vi "READ Configurations V1.00.vi"(2 "OpenParameters(T)orDataBuffers(F)":bool, 6 "CCD Scan Parameters.INI path":path, 9 "CCD Scan Parameters.Data path":path) -> (0 "Parameters":T2={"Magnetic Field"=0.0, "Temperature"=0.0, "Exposure Time"=0.0, "Mag ID string"="Cell 12", "User Name"="Albert Einstein", "Comments"="", "SaveComments?"=1, "X-Axis Unit"=1, "Delimiter"=0, "File Format"=0, "Sample Name"="Sample1"} {"File Format" items=["Macintosh (EOL: CR)", "Unix (EOL: LF)", "DOS/Windows (EOL: CR+LF)"]; "Delimiter" items=["TAB", "COMMA", "SPACE"]; "X-Axis Unit" items=["Point #", "nm", "eV", "meV", "cm-1"]; "SaveComments?" items=["Bare data only", "Saved in the Header Area", "Saved as a Parameter File"]; "Exposure Time" format="%.2f"; "Temperature" format="%.2f"; "Magnetic Field" format="%.2f"}, 1 "Parameters#2":T3={"MaxBufferSize"=2, "Mag GPIB Address"=5, "Max Current (kA)"=36.0, "LTC-GPIB Address"="", "Temp Tolerance"=1.0} {"Temp Tolerance" format="%.2f"; "Max Current (kA)" format="%.2f"}, 3 "X-Axis Array":dbl[][](array[numeric]) format="%.2f", 4 "Data Array":dbl[][](array[numeric]) format="%.2f", 5 "Control Parameters":T1={"Grating Density"=enum."1200", "Offset"=0.0, "Save All Data in ONE file"=FALSE, "Auto Save Data"=FALSE, "Most recent saved file"=path "erererere", "Filename Prefix"="MyData", "Extension"=4, "Suffix"="", "Current Path"=path "/Volumes/DATA"} {"Extension" items=["DOS field", "\".001\",\".002\", ...", "001 (No dot)", "\".A\",\".B\", ...", "±Field", "pField nField", "Temperature", "User Defined"]; "Offset" format="%.2f"}, 7 "Background":i32[](array[numeric])=[1198, 1190, 1193, 1194, 1189, 1188, 1196, 1190, 1202, 1191, 1193, 1192, 1199, 1189, 1194, 1189, 1197, 1191, 1187, 1192, 1195, 1189, 1195, 1191, 1199, 1194, 1192, 1191, 1193, 1197, 1193, 1193, 1194, 1200, 1191, 1190, 1187, 1195, 1189, 1188, 1191, 1194, 1187, 1192, 1198, 1193, 1190, 1192, 1190, 1193, 1191, 1190, 1191, 1189, 1192, 1194, 1190, 1193, 1193, 1191, 1194, 1182, 1190, 1188, 1199, 1192, 1196, 1195, 1186, 1189, 1188, 1185, 1194, 1187, 1193, 1194, 1190, 1189, 1189, 1187, 1196, 1195, 1191, 1197, 1192, 1200, 1187, 1194, 1189, 1193, 1195, 1196, 1186, 1192, 1190, 1194, 1194, 1190, 1191, 1193, 1197, 1197, 1185, 1199, 1190, 1195, 1196, 1184, 1193, 1193, 1193, 1191, 1189, 1190, 1199, 1193, 1191, 1194, 1191, 1192, 1186, 1190, 1194, 1189, 1194, 1190, 1191, 1192, 1192, 1196, 1192, 1192, 1189, 1193, 1198, 1186, 1191, 1193, 1187, 1194, 1190, 1190, 1191, 1189, 1194, 1195, 1189, 1192, 1185, 1193, 1192, 1192, 1189, 1191, 1191, 1190, 1196, 1194, 1193, 1191, 1189, 1191, 1196, 1192, 1192, 1189, 1196, 1191, 1193, 1192, 1188, 1190, 1194, 1192, 1185, 1191, 1194, 1191, 1189, 1195, 1192, 1196, 1190, 1193, 1191, 1189, 1194, 1195, 1191, 1187, 1190, 1196, 1196, 1192, 1197, 1191, 1189, 1192, 1192, 1200, 1192, 1193, 1190, 1192, 1187, 1198, 1186, 1196, 1201, 1199, 1200, 1191, 1196, 1200, 1192, 1191, 1193, 1185, 1192, 1194, 1186, 1190, 1188, 1189, 1201, 1197, 1191, 1194, 1193, 1194, 1195, 1198, 1200, 1192, 1192, 1193, 1193, 1195, 1187, 1193, 1192, 1187, 1189, 1186, 1191, 1197, 1191, 1200, 1194, 1192, 1187, 1196, 1191, 1191, 1196, 1187, 1190, 1193, 1189, 1193, 1190, 1188, 1188, 1190, 1197, 1188, 1191, 1195, 1188, 1191, 1188, 1194, 1193, 1187, 1200, 1192, 1197, 1190, 1196, 1200, 1191, 1189, 1193, 1189, 1186, 1196, 1185, 1198, 1195, 1186, 1191, 1197, 1191, 1193, 1195, 1193, 1191, 1198, 1189, 1183, 1200, 1197, 1192, 1192, 1192, 1196, 1191, 1190, 1194, 1188, 1198, 1193, 1195, 1190, 1187, 1192, 1191, 1195, 1188, 1190, 1191, 1187, 1189, 1185, 1189, 1196, 1198, 1191, 1190, 1196, 1197, 1193, 1187, 1186, 1195, 1191, 1193, 1192, 1196, 1190, 1192, 1192, 1192, 1190, 1195, 1192, 1191, 1193, 1197, 1184, 1190, 1188, 1192, 1194, 1190, 1193, 1195, 1195, 1194, 1189, 1193, 1191, 1194, 1186, 1189, 1192, 1191, 1182, 1190, 1197, 1194, 1188, 1193, 1191, 1186, 1194, 1197, 1193, 1191, 1187, 1194, 1194, 1191, 1189, 1195, 1194, 1189, 1196, 1187, 1186, 1192, 1194, 1196, 1191, 1193, 1191, 1188, 1190, 1199, 1198, 1196, 1196, 1190, 1194, 1191, 1194, 1187, 1195, 1190, 1194, 1196, 1194, 1189, 1193, 1189, 1194, 1189, 1195, 1192, 1194, 1193, 1191, 1197, 1187, 1189, 1189, 1188, 1197, 1192, 1189, 1193, 1194, 1183, 1202, 1187, 1192, 1184, 1188, 1186, 1193, 1189, 1195, 1189, 1193, 1197, 1189, 1194, 1191, 1194, 1192, 1191, 1191, 1196, 1194, 1190, 1193, 1192, 1195, 1197, 1198, 1193, 1202, 1196, 1194, 1194, 1190, 1193, 1190, 1195, 1192, 1187, 1194, 1197, 1190, 1194, 1189, 1198, 1192, 1191, 1192, 1192, 1191, 1191, 1193, 1191, 1191, 1198, 1186, 1192, 1185, 1185, 1188, 1194, 1196, 1194, 1195, 1190, 1194, 1191, 1190, 1195, 1191, 1191, 1195, 1192, 1194, 1201, 1187, 1191, 1195, 1187, 1192, 1192, 1193, 1200, 1188, 1189, 1189, 1197, 1189, 1188, 1197, 1195, 1191, 1189, 1190, 1195, 1189, 1191, 1194, 1186, 1192, 1190, 1191, 1188, 1195, 1192, 1191, 1191, 1199, 1190, 1190, 1190, 1192, 1187, 1193, 1197, 1197, 1186, 1193, 1189, 1192, 1197, 1184, 1187, 1188, 1192, 1192, 1192, 1189, 1192, 1190, 1194, 1191, 1186, 1196, 1194, 1189, 1193, 1191, 1186, 1189, 1193, 1195, 1196, 1197, 1199, 1194, 1190, 1193, 1194, 1190, 1198, 1196, 1194, 1195, 1194, 1184, 1188, 1195, 1197, 1190, 1194, 1190, 1191, 1195, 1198, 1188, 1193, 1194, 1195, 1198, 1195, 1191, 1197, 1192, 1198, 1190, 1196, 1191, 1194, 1188, 1189, 1198, 1192, 1198, 1195, 1185, 1191, 1193, 1192, 1197, 1195, 1195, 1195, 1193, 1190, 1190, 1190, 1198, 1195, 1191, 1194, 1190, 1190, 1194, 1194, 1195, 1192, 1190, 1194, 1195, 1192, 1192, 1194, 1189, 1192, 1193, 1188, 1194, 1195, 1196, 1193, 1192, 1201, 1191, 1198, 1197, 1191, 1192, 1191, 1194, 1193, 1188, 1192, 1189, 1183, 1189, 1190, 1192, 1189, 1196, 1193, 1197, 1185, 1193, 1189, 1191, 1196, 1195, 1193, 1193, 1191, 1189, 1193, 1192, 1192, 1192, 1190, 1191, 1193, 1193, 1197, 1195, 1189, 1193, 1188, 1194, 1197, 1194, 1195, 1196, 1190, 1194, 1188, 1197, 1195, 1191, 1195, 1192, 1194, 1188, 1190, 1197, 1197, 1191, 1187, 1197, 1191, 1193, 1188, 1191, 1194, 1193, 1195, 1192, 1195, 1189, 1193, 1193, 1195, 1190, 1192, 1196, 1188, 1187, 1193, 1192, 1192, 1194, 1185, 1199, 1190, 1193, 1191, 1198, 1189, 1190, 1191, 1190, 1193, 1195, 1186, 1190, 1193, 1191, 1189, 1197, 1193, 1198, 1190, 1192, 1193, 1191, 1196, 1193, 1196, 1190, 1190, 1198, 1192, 1199, 1198, 1190, 1191, 1191, 1196, 1190, 1196, 1195, 1191, 1196, 1195, 1193, 1190, 1190, 1195, 1193, 1187, 1197, 1185, 1191, 1189, 1191, 1193, 1192, 1188, 1196, 1193, 1191, 1193, 1193, 1190, 1192, 1192, 1192, 1195, 1191, 1195, 1189, 1189, 1191, 1191, 1185, 1192, 1191, 1193, 1201, 1199, 1197, 1206, 1201, 1207, 1200, 1198, 1195, 1188, 1194, 1186, 1190, 1197, 1188, 1193, 1196, 1193, 1192, 1192, 1188, 1196, 1186, 1193, 1194, 1188, 1190, 1190, 1192, 1190, 1191, 1191, 1200, 1192, 1199, 1193, 1190, 1190, 1199, 1187, 1193, 1190, 1188, 1194, 1194, 1196, 1194, 1195, 1190, 1187, 1187, 1196, 1193, 1199, 1190, 1193, 1193, 1191, 1198, 1192, 1193, 1192, 1193, 1189, 1189, 1197, 1189, 1194, 1193, 1192, 1185, 1198, 1193, 1189, 1192, 1193, 1196, 1190, 1195, 1189, 1196, 1198, 1190, 1191, 1193, 1186, 1189, 1195, 1188, 1197, 1188, 1191, 1185, 1190, 1193, 1188, 1198, 1192, 1193, 1194, 1194, 1189, 1184, 1193, 1199, 1193, 1192, 1193, 1190, 1196, 1191, 1192, 1189, 1194, 1188, 1189, 1190, 1190, 1192, 1195, 1188, 1190, 1192, 1189, 1197, 1192, 1194, 1187, 1196, 1192, 1194, 1185, 1187, 1187, 1191, 1195, 1190, 1186, 1183, 1194, 1194, 1192, 1192, 1188, 1193, 1195, 1189, 1190, 1191, 1192, 1196, 1186, 1195, 1191, 1185, 1191, 1187, 1190, 1188, 1189, 1187, 1196, 1191, 1190, 1191, 1190, 1196, 1195, 1186, 1187, 1187, 1188, 1194, 1192, 1192, 1192, 1189, 1192, 1191, 1188, 1188, 1187, 1187, 1190, 1186, 1191, 1195, 1192, 1196, 1193, 1192, 1191, 1189, 1187, 1193, 1188, 1189, 1194, 1191, 1185, 1193, 1191, 1196, 1196, 1199, 1195, 1211], 8 "FieldRamp Parameters":dbl[][](array[numeric])=[[0.0, 30.0, 1.0, 400.0], [30.0, 0.0, -1.0, 400.0], [0.0, -30.0, -1.0, 400.0], [-30.0, 0.0, 1.0, 400.0], [0.0, 30.0, 0.5, 200.0], [30.0, 0.0, -0.5, 200.0]] step=1.0 format="%.2f")   [LabVIEW 2025]
doc: "Author: Scott Hannahs <sth@magnet.fsu.edu>\n\nThis software is licensed for use under the “MIT License\"\nCopyright (c) 2025 Scott Hannahs, sth@sth@magnet.sthnet.net\n\nPermission is hereby granted, free of charge, to any person obtaining a copy of this software and associated documentation files (the \"Software\"), to deal in the Software without restriction, including without limitation the rights to use, copy, modify, merge, publish, distribute, sublicense, and/or sell copies of the Software, and to permit persons to whom the Software is furnished to do so, subject to the following conditions: The above copyright notice and this permission notice shall be included in all copies or substantial portions of the Software.\n\nTHE SOFTWARE IS PROVIDED \"AS IS\", WITHOUT WARRANTY OF ANY KIND, EXPRESS OR IMPLIED, INCLUDING BUT NOT LIMITED TO THE WARRANTIES OF MERCHANTABILITY, FITNESS FOR A PARTICULAR PURPOSE AND NONINFRINGEMENT. IN NO EVENT SHALL THE AUTHORS OR COPYRIGHT HOLDERS BE LIABLE FOR ANY CLAIM, DAMAGES OR OTHER LIABILITY, WHETHER IN AN ACTION OF CONTRACT, TORT OR OTHERWISE, ARISING FROM, OUT OF OR IN CONNECTION WITH THE SOFTWARE OR THE USE OR OTHER DEALINGS IN THE SOFTWARE."
uses:
  Parameters#2.ctl
  Parameters#1.ctl
  Parameters_Control.ctl
  <vilib>/Utility/config.llb/Read Key (String).vi
  <vilib>/Utility/config.llb/Read Key (U32).vi
  <vilib>/Utility/config.llb/Read Key (Double).vi
  <vilib>/Utility/config.llb/Read Key (Boolean).vi
  <vilib>/Utility/config.llb/Read Key (Path).vi
  <vilib>/Utility/config.llb/NI_LVConfig.lvlib
panel:
  out "Temperature array":sgl[](array[numeric]) format="%.3f"
  out "Field array":sgl[](array[numeric]) format="%.3f"
  out "2D Y-array":sgl[][](array[numeric]) format="%.3f"
  out "2D X-array":sgl[][](array[numeric]) format="%.3f"
  out "error out":errorcluster
  out "found?":bool
  out "Buffer Size":i32[](array[numeric])
  out "FieldRampSize":i32[](array[numeric])
  out "X-size":i32[](array[numeric])
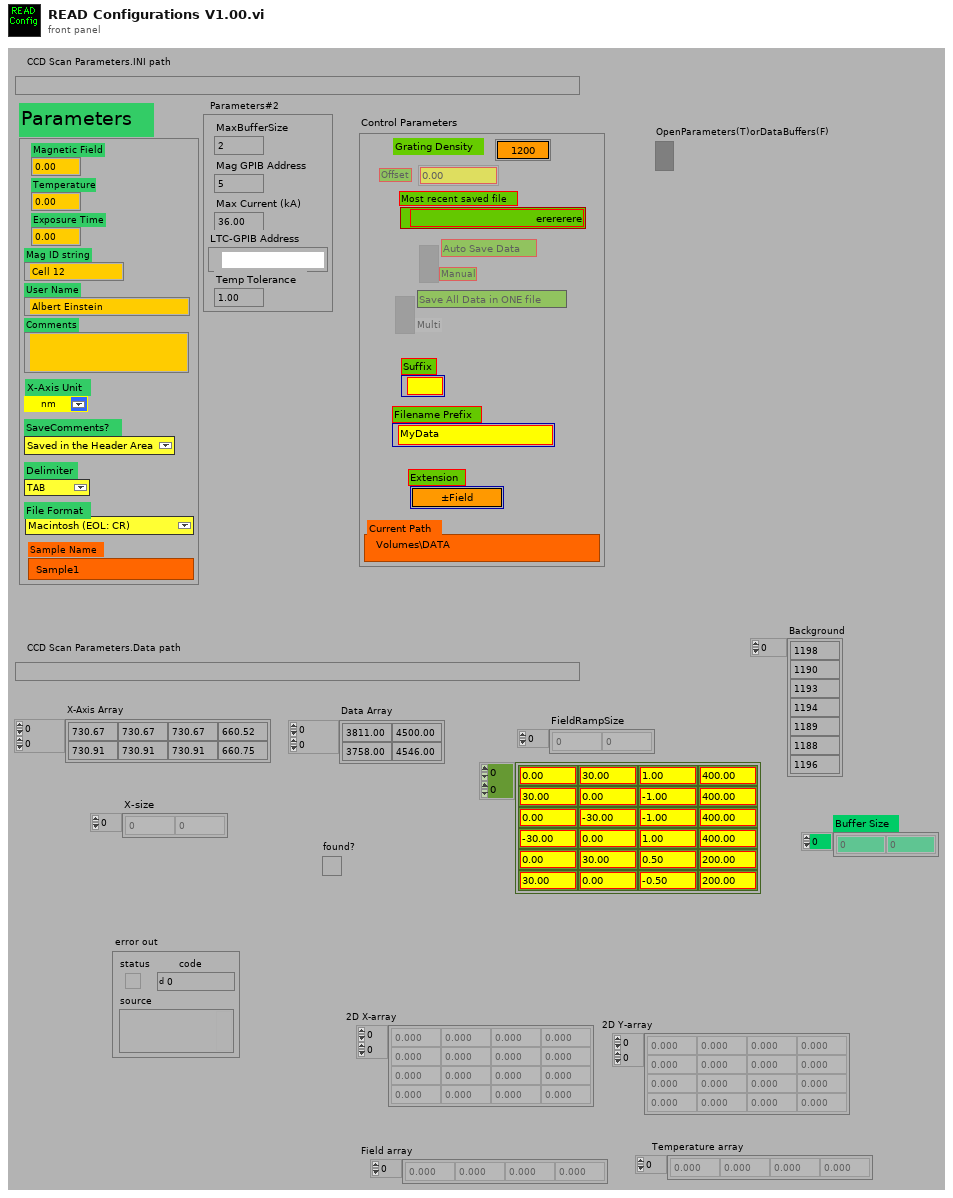
[diagram p1: front panel]
types:
  T1 = typedef "Parameters_Control.ctl" = cluster{"Grating Density":enum16{"150", "300", "600", "1200", "1800"}, "Offset":dbl, "Save All Data in ONE file":bool, "Auto Save Data":bool, "Most recent saved file":path, "Filename Prefix":string, "Extension":u16, "Suffix":string, "Current Path":path}
  T2 = typedef "Parameters#1.ctl" = cluster{"Magnetic Field":dbl, "Temperature":dbl, "Exposure Time":dbl, "Mag ID string":string, "User Name":string, "Comments":string, "SaveComments?":u16, "X-Axis Unit":u16, "Delimiter":u16, "File Format":u16, "Sample Name":string}
  T3 = typedef "Parameters#2.ctl" = cluster{"MaxBufferSize":i32, "Mag GPIB Address":i32, "Max Current (kA)":dbl, "LTC-GPIB Address":refnum<visa-resource-name>, "Temp Tolerance":dbl}
  T4 = typedef "NI_LVConfig.lvlib/Config Data RefNum.ctl" = refnum<k1>
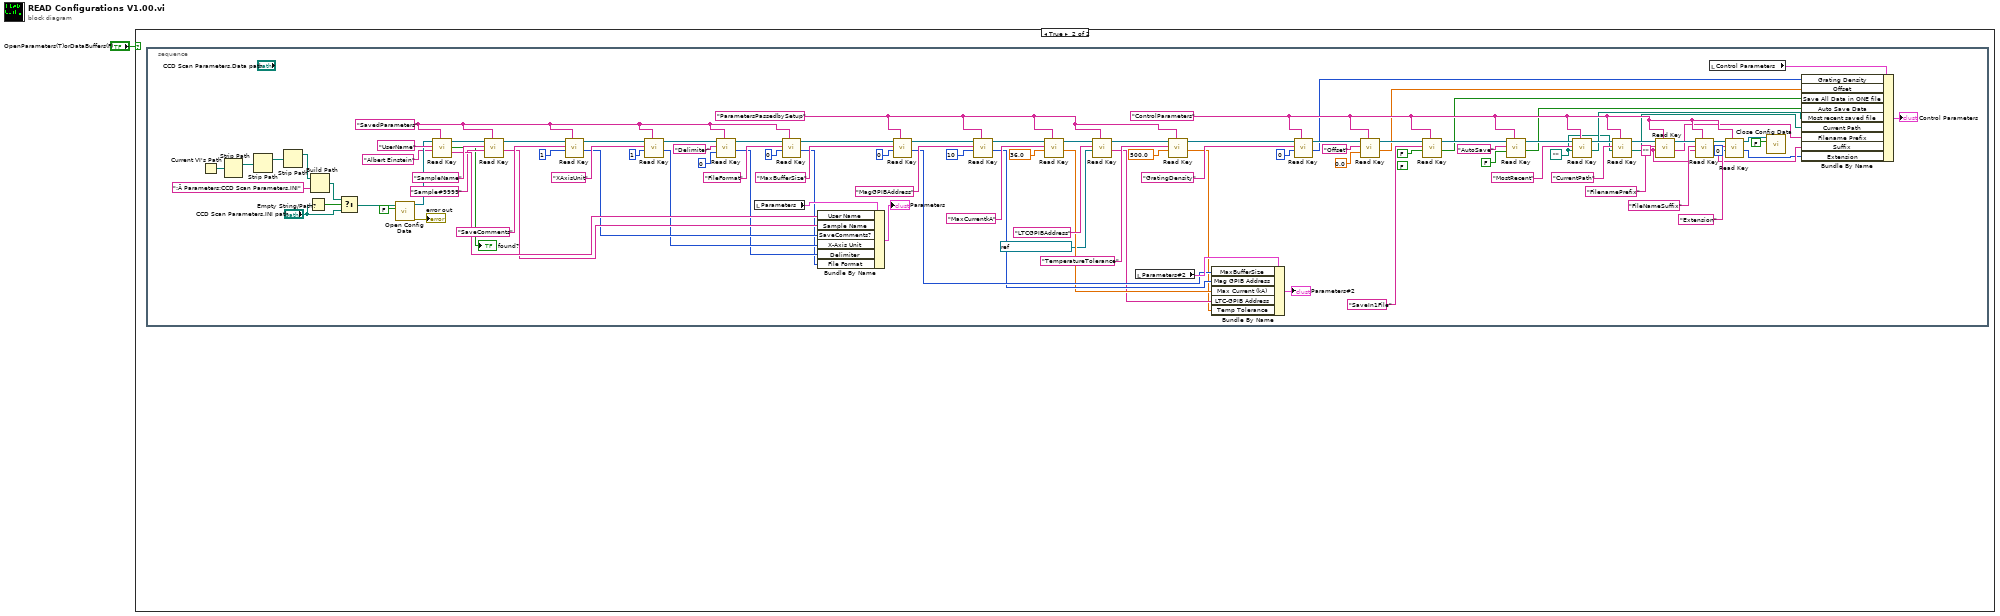
[diagram p0: block diagram]
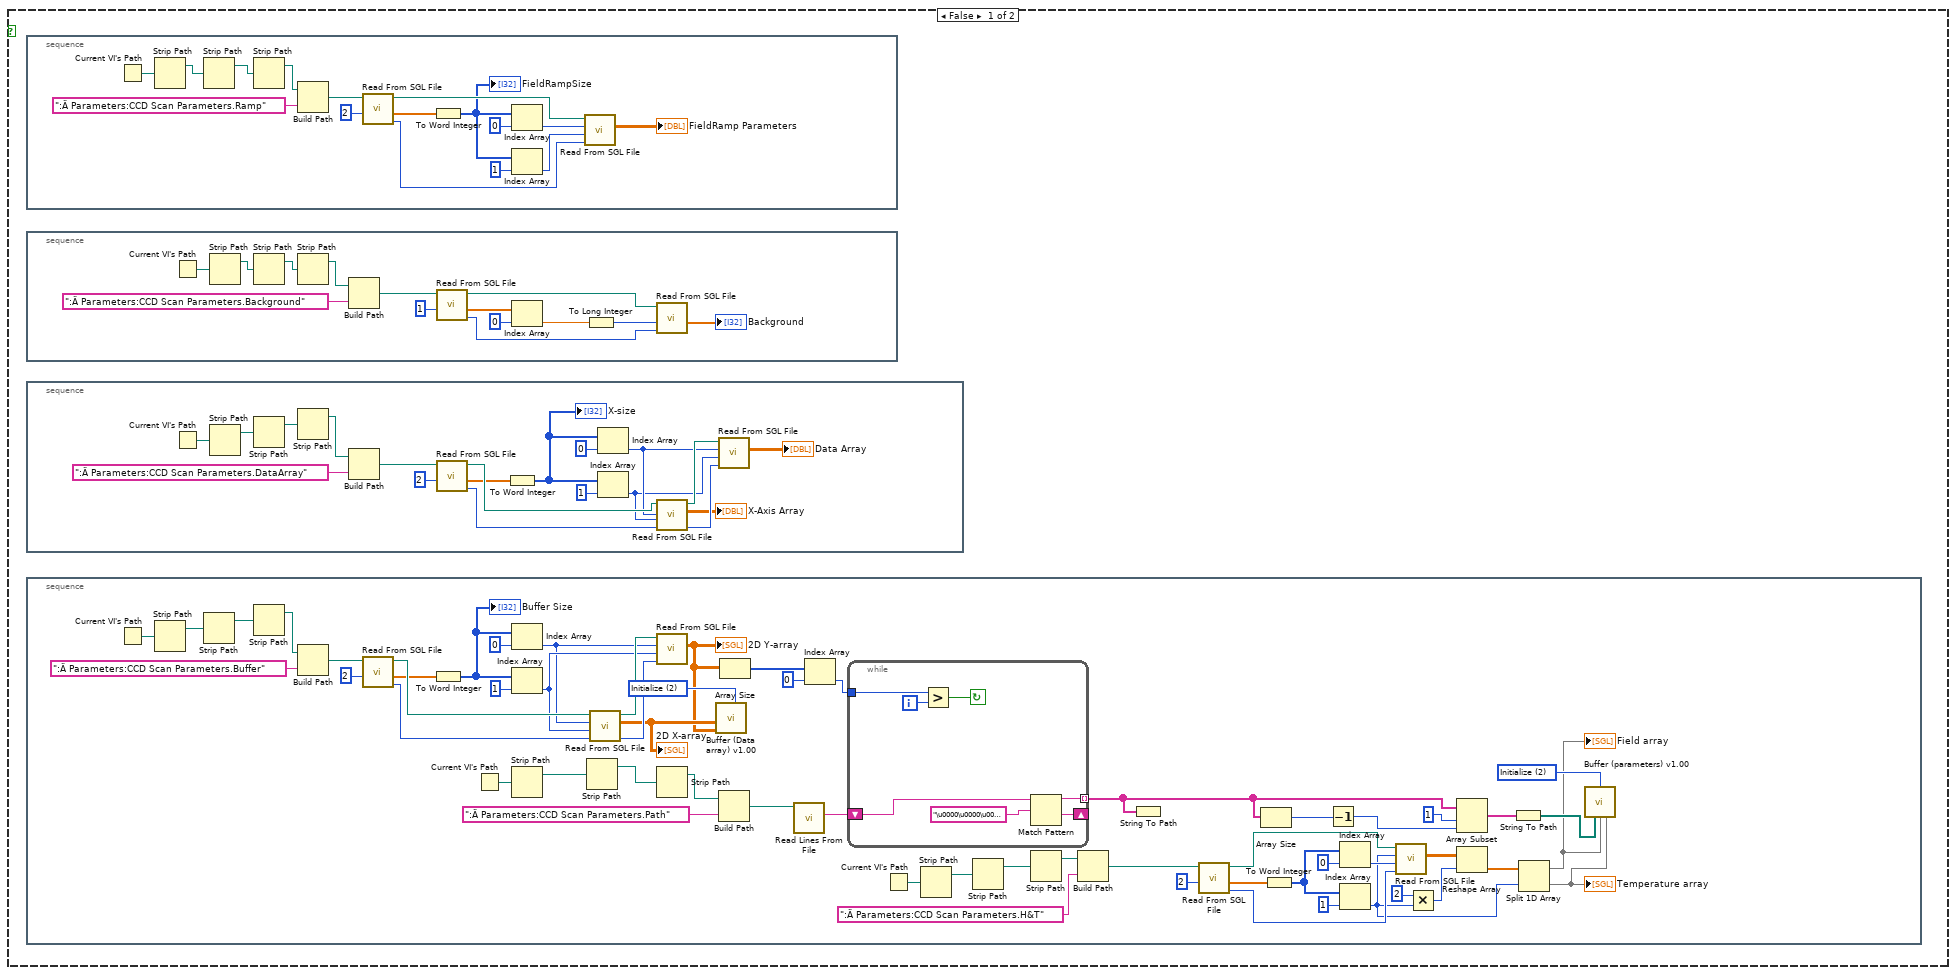
[diagram p2: hidden frame]
diagram:
  n1 = case shown="True" "OpenParameters(T)orDataBuffers(F)" {
    frame False {
      n2 = stacked-sequence {
        frame #0 {
          n3 = Current VI's Path() -> (path=w18:path)
          n4 = Strip Path(path=w18) -> (stripped path=w22:path)  [unwired: 1 out]
          n5 = Strip Path(path=w22) -> (stripped path=w21:path)  [unwired: 1 out]
          n6 = Strip Path(path=w21) -> (stripped path=w19:path)  [unwired: 1 out]
          n7 = Build Path(base path=w19, name or relative path=":Ä Parameters:CCD Scan Parameters.Ramp") -> (appended path=w17:path)
          n8 = call <vilib>:"Read From SGL File.vi"("2D number of columns/1D count (all as 1D: -1)"=2, "file path (dialog if empty)"=w17) -> ("mark after read (bytes)"=w30:i32, "1D array"=w26:sgl[], "new file path (Not A Path if cancelled)"=w31:path)  [unwired: 5 in, 2 out]
          n9 = To Word Integer(number=w26) -> (16bit integer=w23:i16[])
          "FieldRampSize" <- w23
          n10 = Index Array(array=w23, index=0) -> (element=w25:i16)
          n11 = Index Array(array=w23, index=1) -> (element=w24:i16)
          n12 = call <vilib>:"Read From SGL File.vi"("start of read offset (bytes:0)"=w30, "2D number of columns/1D count (all as 1D: -1)"=w24, "2D number of rows"=w25, "file path (dialog if empty)"=w31) -> ("2D array"=→"FieldRamp Parameters":sgl[][])  [unwired: 3 in, 4 out]
        }
      }
      n13 = stacked-sequence {
        frame #0 {
          n14 = Current VI's Path() -> (path=w3:path)
          n15 = Strip Path(path=w3) -> (stripped path=w7:path)  [unwired: 1 out]
          n16 = Strip Path(path=w7) -> (stripped path=w6:path)  [unwired: 1 out]
          n17 = Strip Path(path=w6) -> (stripped path=w4:path)  [unwired: 1 out]
          n18 = Build Path(base path=w4, name or relative path=":Ä Parameters:CCD Scan Parameters.Background") -> (appended path=w2:path)
          n19 = call <vilib>:"Read From SGL File.vi"("2D number of columns/1D count (all as 1D: -1)"=1, "file path (dialog if empty)"=w2) -> ("mark after read (bytes)"=w12:i32, "1D array"=w14:sgl[], "new file path (Not A Path if cancelled)"=w11:path)  [unwired: 5 in, 2 out]
          n20 = Index Array(array=w14, index=0) -> (element=w10:sgl)
          n21 = To Long Integer(number=w10) -> (32bit integer=w9:i32)
          n22 = call <vilib>:"Read From SGL File.vi"("start of read offset (bytes:0)"=w12, "2D number of columns/1D count (all as 1D: -1)"=w9, "file path (dialog if empty)"=w11) -> ("1D array"=→"Background":sgl[])  [unwired: 4 in, 4 out]
        }
      }
      n23 = stacked-sequence {
        frame #0 {
          n24 = Current VI's Path() -> (path=w46:path)
          n25 = Strip Path(path=w46) -> (stripped path=w50:path)  [unwired: 1 out]
          n26 = Strip Path(path=w50) -> (stripped path=w49:path)  [unwired: 1 out]
          n27 = Strip Path(path=w49) -> (stripped path=w47:path)  [unwired: 1 out]
          n28 = Build Path(base path=w47, name or relative path=":Ä Parameters:CCD Scan Parameters.DataArray") -> (appended path=w32:path)
          n29 = call <vilib>:"Read From SGL File.vi"("2D number of columns/1D count (all as 1D: -1)"=2, "file path (dialog if empty)"=w32) -> ("mark after read (bytes)"=w43:i32, "1D array"=w40:sgl[], "new file path (Not A Path if cancelled)"=w44:path)  [unwired: 5 in, 2 out]
          n30 = To Word Integer(number=w40) -> (16bit integer=w33:i16[])
          "X-size" <- w33
          n31 = Index Array(array=w33, index=0) -> (element=w36:i16)
          n32 = Index Array(array=w33, index=1) -> (element=w35:i16)
          n33 = call <vilib>:"Read From SGL File.vi"("start of read offset (bytes:0)"=w43, "2D number of columns/1D count (all as 1D: -1)"=w35, "2D number of rows"=w36, "file path (dialog if empty)"=w44) -> ("mark after read (bytes)"=w42:i32, "2D array"=→"X-Axis Array":sgl[][], "new file path (Not A Path if cancelled)"=w45:path)  [unwired: 3 in, 2 out]
          n34 = call <vilib>:"Read From SGL File.vi"("start of read offset (bytes:0)"=w42, "2D number of columns/1D count (all as 1D: -1)"=w35, "2D number of rows"=w36, "file path (dialog if empty)"=w45) -> ("2D array"=→"Data Array":sgl[][])  [unwired: 3 in, 4 out]
        }
      }
      n35 = stacked-sequence {
        frame #0 {
          w96 = u16 2 items=["Read", "Write", "Initialize"] ("Read(0) or Write(1)")
          w99 = u16 2 items=["Read", "Write", "Initialize"] ("Read(0) or Write(1)")
          n36 = Current VI's Path() -> (path=w80:path)
          n37 = Strip Path(path=w80) -> (stripped path=w84:path)  [unwired: 1 out]
          n38 = Strip Path(path=w84) -> (stripped path=w83:path)  [unwired: 1 out]
          n39 = Strip Path(path=w83) -> (stripped path=w81:path)  [unwired: 1 out]
          n40 = Build Path(base path=w81, name or relative path=":Ä Parameters:CCD Scan Parameters.Buffer") -> (appended path=w79:path)
          n41 = call <vilib>:"Read From SGL File.vi"("2D number of columns/1D count (all as 1D: -1)"=2, "file path (dialog if empty)"=w79) -> ("mark after read (bytes)"=w106:i32, "1D array"=w101:sgl[], "new file path (Not A Path if cancelled)"=w108:path)  [unwired: 5 in, 2 out]
          n42 = To Word Integer(number=w101) -> (16bit integer=w97:i16[])
          "Buffer Size" <- w97
          n43 = Current VI's Path() -> (path=w91:path)
          n44 = Index Array(array=w97, index=0) -> (element=w73:i16)
          n45 = Index Array(array=w97, index=1) -> (element=w100:i16)
          n46 = Strip Path(path=w91) -> (stripped path=w95:path)  [unwired: 1 out]
          n47 = Strip Path(path=w95) -> (stripped path=w94:path)  [unwired: 1 out]
          n48 = call <vilib>:"Read From SGL File.vi"("start of read offset (bytes:0)"=w106, "2D number of columns/1D count (all as 1D: -1)"=w100, "2D number of rows"=w73, "file path (dialog if empty)"=w108) -> ("mark after read (bytes)"=w105:i32, "2D array"=w98:sgl[][], "new file path (Not A Path if cancelled)"=w107:path)  [unwired: 3 in, 2 out]
          "2D X-array" <- w98
          n49 = call <vilib>:"Read From SGL File.vi"("start of read offset (bytes:0)"=w105, "2D number of columns/1D count (all as 1D: -1)"=w100, "2D number of rows"=w73, "file path (dialog if empty)"=w107) -> ("2D array"=w63:sgl[][])  [unwired: 3 in, 4 out]
          "2D Y-array" <- w63
          n50 = Strip Path(path=w94) -> (stripped path=w92:path)  [unwired: 1 out]
          n51 = call "Buffer (Data array) v1.00.vi"("Action"=w99, "Y-Buffer input"=w63, "X-Buffer input"=w98) -> ()  [unwired: 5 in, 4 out]
          n52 = Build Path(base path=w92, name or relative path=":Ä Parameters:CCD Scan Parameters.Path") -> (appended path=w90:path)
          n53 = Array Size(array=w63) -> (size(s)=w62:i32[])
          n54 = call <vilib>:"Read Lines From File.vi"("file path (dialog if empty)"=w90) -> ("line string"=w89:string)  [unwired: 5 in, 3 out]
          n55 = Index Array(array=w62, index=0 ("Index")) -> (element=w58:i32)
          n56 = while {
            tunnel: w58 -> [w109]
            tunnel: [w112] -> w60 mode=indexing
            shift-left: w89 -> [w114]
            shift-right: [w113] -> _
            i -> [w110]
            stop <- w111 continue-if-true
            n57 = Greater?(x=w109, y=w110) -> (0:w111:bool)
            n58 = Match Pattern(string=w114, regular expression="\u0000\u0000\u0000\u001d") -> (before substring=w112:string, after substring=w113:string)  [unwired: 1 in, 2 out]
          }
          n59 = Current VI's Path() -> (path=w75:path)
          n60 = Strip Path(path=w75) -> (stripped path=w78:path)  [unwired: 1 out]
          n61 = Strip Path(path=w78) -> (stripped path=w77:path)  [unwired: 1 out]
          n62 = Strip Path(path=w77) -> (stripped path=w76:path)  [unwired: 1 out]
          n63 = Build Path(base path=w76, name or relative path=":Ä Parameters:CCD Scan Parameters.H&T") -> (appended path=w67:path)
          n64 = String To Path(string=w60) -> ()  [unwired: 1 out]
          n65 = call <vilib>:"Read From SGL File.vi"("2D number of columns/1D count (all as 1D: -1)"=2, "file path (dialog if empty)"=w67) -> ("mark after read (bytes)"=w65:i32, "1D array"=w69:sgl[], "new file path (Not A Path if cancelled)"=w66:path)  [unwired: 5 in, 2 out]
          n66 = Array Size(array=w60) -> (size(s)=w86:i32)
          n67 = To Word Integer(number=w69) -> (16bit integer=w68:i16[])
          n68 = Decrement(x=w86) -> (x-1=w88:i32)
          n69 = Index Array(array=w68, index=0) -> (element=w64:i16)
          n70 = Index Array(array=w68, index=1) -> (element=w51:i16)
          n71 = call <vilib>:"Read From SGL File.vi"("start of read offset (bytes:0)"=w65, "2D number of columns/1D count (all as 1D: -1)"=w64, "2D number of rows"=w51, "file path (dialog if empty)"=w66) -> ("2D array"=w57:sgl[][])  [unwired: 3 in, 4 out]
          n72 = Multiply(x=i16 2, y=w51) -> (x*y=w55:i16)
          n73 = Array Subset(array=w60, index=1, length=w88) -> (w85:string[])
          n74 = Reshape Array(w57, w55) -> (w54:sgl[])
          n75 = String To Path(string=w85) -> (path=w59:path[])
          n76 = Split 1D Array(array=w54, index=w51) -> (first subarray=w53:sgl[], second subarray=w52:sgl[])
          "Field array" <- w53
          "Temperature array" <- w52
          n77 = call "Buffer (parameters) v1.00.vi"("Action"=w96, "FilePath Buffer in"=w59, "Field Buffer in"=w53, "Temperature Buffer in"=w52) -> ()  [unwired: 7 in, 5 out]
        }
      }
    }
    frame True {
      n78 = stacked-sequence {
        frame #0 {
          w117 = "" ("default value")
          w118 = path "" ("default value")
          (unwired) FALSE ("write configuration file? (T)")
          w163 = "ControlParameters" ("section")
          w185 = "ParametersPassedbySetup" ("section")
          w196 = "SavedParameters" ("section")
          n79 = Current VI's Path() -> (path=w210:path)
          n80 = Strip Path(path=w210) -> (stripped path=w215:path)  [unwired: 1 out]
          n81 = Strip Path(path=w215) -> (stripped path=w214:path)  [unwired: 1 out]
          n82 = Strip Path(path=w214) -> (stripped path=w211:path)  [unwired: 1 out]
          n83 = Empty String/Path?(string/path="CCD Scan Parameters.INI path") -> (empty?=w216:bool)
          n84 = Build Path(base path=w211, name or relative path=":Ä Parameters:CCD Scan Parameters.INI") -> (appended path=w209:path)
          n85 = Select(t=w209, s=w216, f="CCD Scan Parameters.INI path") -> (s? t:f=w208:path)
          n86 = call <vilib>:"Open Config Data.vi"("create file if necessary (T)"=FALSE ("create file if necessary? (T)"), "configuration file path"=w208) -> ("error out"=→"error out":errorcluster, "refnum"=w184:T4)  [unwired: 7 in, 1 out]
          n87 = call-poly <vilib>:"Read Key.vi"("section"=w196, "default value"="Albert Einstein", "key"="UserName", "refnum"=w184) -> ("value"=w160:string, "found?"=→"found?":bool, "refnum out"=w199:T4)  [unwired: 4 in, 1 out]
          n88 = call-poly <vilib>:"Read Key.vi"("section"=w196, "default value"="Sample#9999", "key"="SampleName", "refnum"=w199) -> ("value"=w159:string, "refnum out"=w198:T4)  [unwired: 4 in, 2 out]
          n89 = call-poly <vilib>:"Read Key.vi"("section"=w196, "default value"=u32 1, "key"="SaveComments", "refnum"=w198) -> ("value"=w158:u32, "refnum out"=w205:T4)  [unwired: 4 in, 2 out]
          n90 = call-poly <vilib>:"Read Key.vi"("section"=w196, "default value"=u32 1, "key"="XAxisUnit", "refnum"=w205) -> ("value"=w157:u32, "refnum out"=w203:T4)  [unwired: 4 in, 2 out]
          n91 = call-poly <vilib>:"Read Key.vi"("section"=w196, "default value"=u32 0, "key"="Delimiter", "refnum"=w203) -> ("value"=w156:u32, "refnum out"=w202:T4)  [unwired: 4 in, 2 out]
          n92 = local read "Parameters"() -> (w161:T2)
          n93 = call-poly <vilib>:"Read Key.vi"("section"=w196, "default value"=u32 0, "key"="FileFormat", "refnum"=w202) -> ("value"=w155:u32, "refnum out"=w195:T4)  [unwired: 4 in, 2 out]
          n94 = Bundle By Name(cluster=w161, "User Name"=w160, "Sample Name"=w159, "SaveComments?"=w158, "X-Axis Unit"=w157, "Delimiter"=w156, "File Format"=w155) -> (→"Parameters":T2)
          n95 = call-poly <vilib>:"Read Key.vi"("section"=w185, "default value"=u32 0, "key"="MaxBufferSize", "refnum"=w195) -> ("value"=w146:u32, "refnum out"=w194:T4)  [unwired: 4 in, 2 out]
          n96 = call-poly <vilib>:"Read Key.vi"("section"=w185, "default value"=u32 10, "key"="MagGPIBAddress", "refnum"=w194) -> ("value"=w145:u32, "refnum out"=w193:T4)  [unwired: 4 in, 2 out]
          n97 = call-poly <vilib>:"Read Key.vi"("section"=w185, "default value"=36.0, "key"="MaxCurrentkA", "refnum"=w193) -> ("value"=w144:dbl, "refnum out"=w192:T4)  [unwired: 4 in, 2 out]
          n98 = call-poly <vilib>:"Read Key.vi"("section"=w185, "default value"=refnum<visa-resource-name> "GPIB0::15::INSTR" ("VISA resource name"), "key"="LTCGPIBAddress", "refnum"=w192) -> ("value"=w143:string, "refnum out"=w191:T4)  [unwired: 4 in, 2 out]
          n99 = local read "Parameters#2"() -> (w148:T3)
          n100 = call-poly <vilib>:"Read Key.vi"("section"=w185, "default value"=500.0, "key"="TemperatureTolerance", "refnum"=w191) -> ("value"=w142:dbl, "refnum out"=w183:T4)  [unwired: 4 in, 2 out]
          n101 = Bundle By Name(cluster=w148, "MaxBufferSize"=w146, "Mag GPIB Address"=w145, "Max Current (kA)"=w144, "LTC-GPIB Address"=w143, "Temp Tolerance"=w142) -> (→"Parameters#2":T3)
          n102 = call-poly <vilib>:"Read Key.vi"("section"=w163, "default value"=u32 0, "key"="GratingDensity", "refnum"=w183) -> ("value"=w136:u32, "refnum out"=w182:T4)  [unwired: 4 in, 2 out]
          n103 = call-poly <vilib>:"Read Key.vi"("section"=w163, "default value"=0.0, "key"="Offset", "refnum"=w182) -> ("value"=w135:dbl, "refnum out"=w181:T4)  [unwired: 4 in, 2 out]
          n104 = call-poly <vilib>:"Read Key.vi"("section"=w163, "default value"=FALSE, "key"="SaveIn1File", "refnum"=w181) -> ("value"=w134:bool, "refnum out"=w180:T4)  [unwired: 4 in, 2 out]
          n105 = call-poly <vilib>:"Read Key.vi"("section"=w163, "default value"=FALSE, "key"="AutoSave", "refnum"=w180) -> ("value"=w133:bool, "refnum out"=w179:T4)  [unwired: 4 in, 2 out]
          n106 = call-poly <vilib>:"Read Key.vi"("section"=w163, "default value"=w118, "key"="MostRecent", "refnum"=w179) -> ("value"=w132:path, "refnum out"=w178:T4)  [unwired: 4 in, 2 out]
          n107 = call-poly <vilib>:"Read Key.vi"("section"=w163, "default value"=w118, "key"="CurrentPath", "refnum"=w178) -> ("value"=w131:path, "refnum out"=w177:T4)  [unwired: 4 in, 2 out]
          n108 = call-poly <vilib>:"Read Key.vi"("section"=w163, "default value"=w117, "key"="FilenamePrefix", "refnum"=w177) -> ("value"=w130:string, "refnum out"=w176:T4)  [unwired: 4 in, 2 out]
          n109 = call-poly <vilib>:"Read Key.vi"("section"=w163, "default value"=w117, "key"="FileNameSuffix", "refnum"=w176) -> ("value"=w129:string, "refnum out"=w175:T4)  [unwired: 4 in, 2 out]
          n110 = local read "Control Parameters"() -> (w137:T1)
          n111 = call-poly <vilib>:"Read Key.vi"("section"=w163, "default value"=u32 0, "key"="Extension", "refnum"=w175) -> ("value"=w128:u32, "refnum out"=w174:T4)  [unwired: 4 in, 2 out]
          n112 = call <vilib>:"Close Config Data.vi"("write file if changed (T)"=FALSE ("write configuration file? (F)"), "refnum"=w174) -> ()  [unwired: 8 in, 2 out]
          n113 = Bundle By Name(cluster=w137, "Grating Density"=w136, "Offset"=w135, "Save All Data in ONE file"=w134, "Auto Save Data"=w133, "Most recent saved file"=w132, "Current Path"=w131, "Filename Prefix"=w130, "Suffix"=w129, "Extension"=w128) -> (→"Control Parameters":T1)
        }
      }
    }
  }
